vi "AO.vi"() -> ()   [LabVIEW 2023]
panel:
  out "error out":errorcluster
  in  "error in (no error)":errorcluster
  out "elements 4":variant[](array[variant])
  out "elements 3":variant[](array[variant])
  out "elements 2":variant[](array[variant])
  out "max queue size":i32
  out "# elements in queue":i32
  out "elements":variant[](array[variant])
  out "current time":timestamp
  out "overflow? 4":bool
  out "overflow? 3":bool
  out "overflow? 2":bool
  out "overflow?":bool
  out "startr_time":timestamp
  out "Waveform Chart":waveform(dbl)(graph)
  in  "Number of Samples":i32=1000
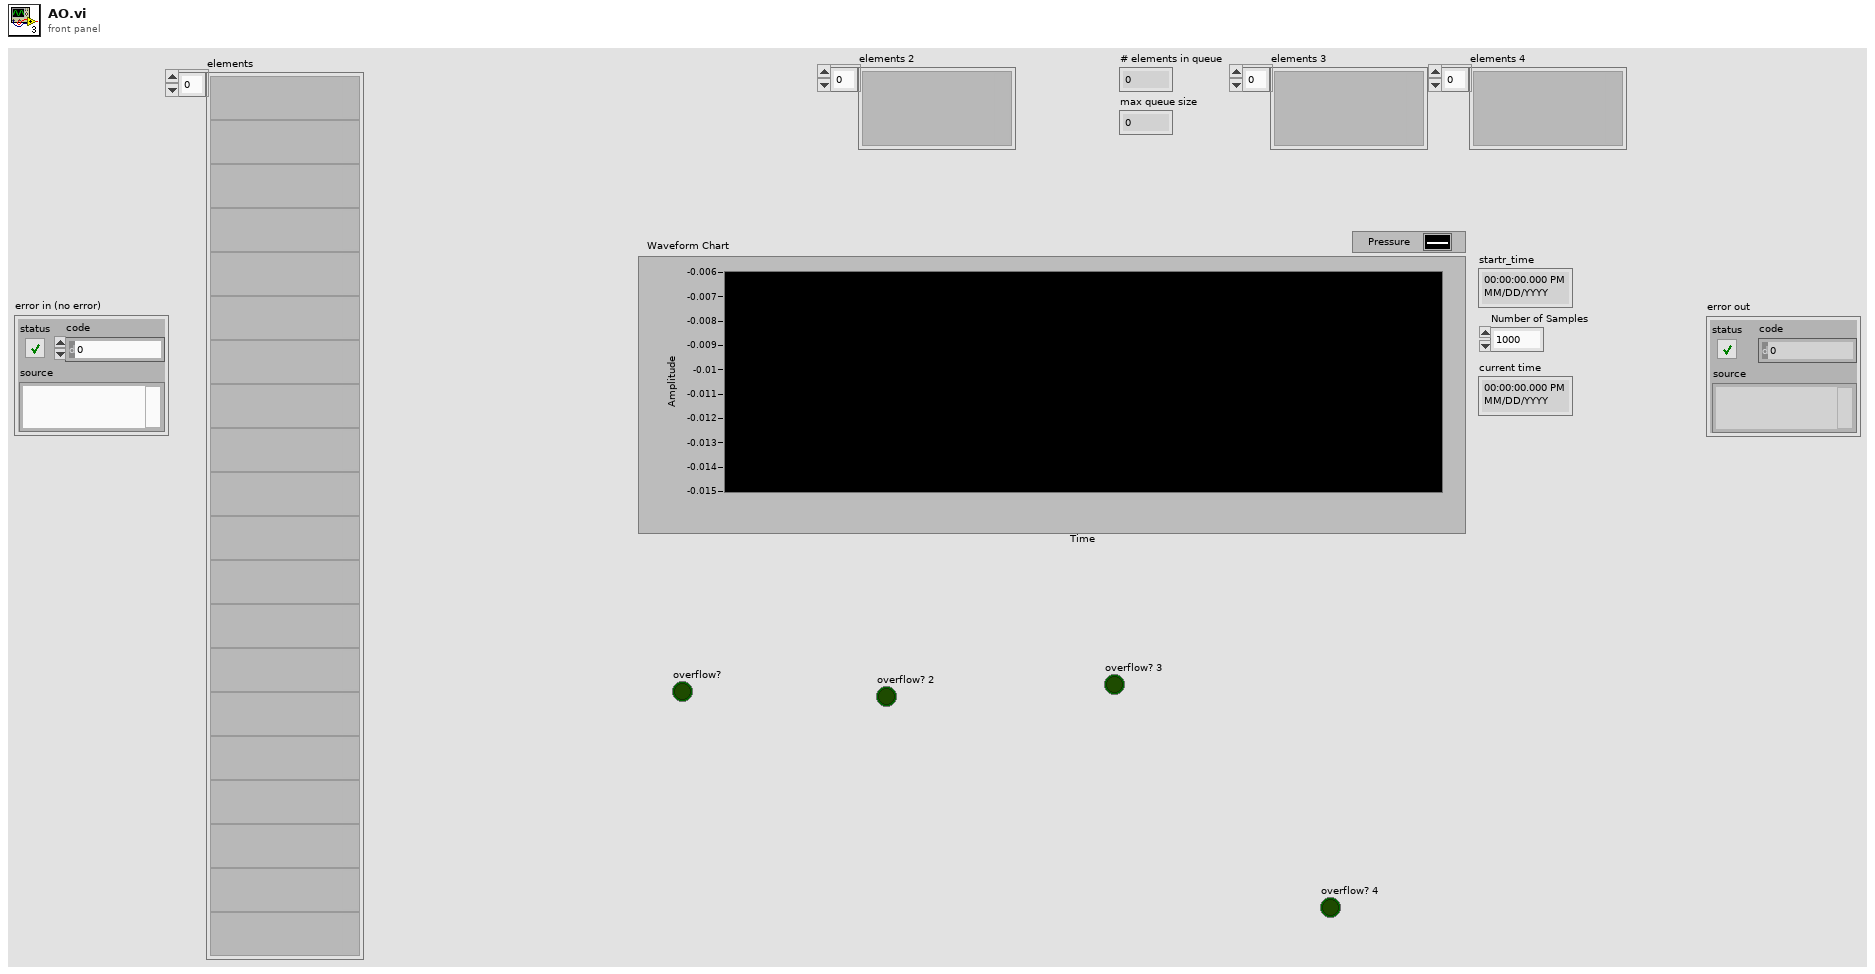
[diagram p1: front panel]
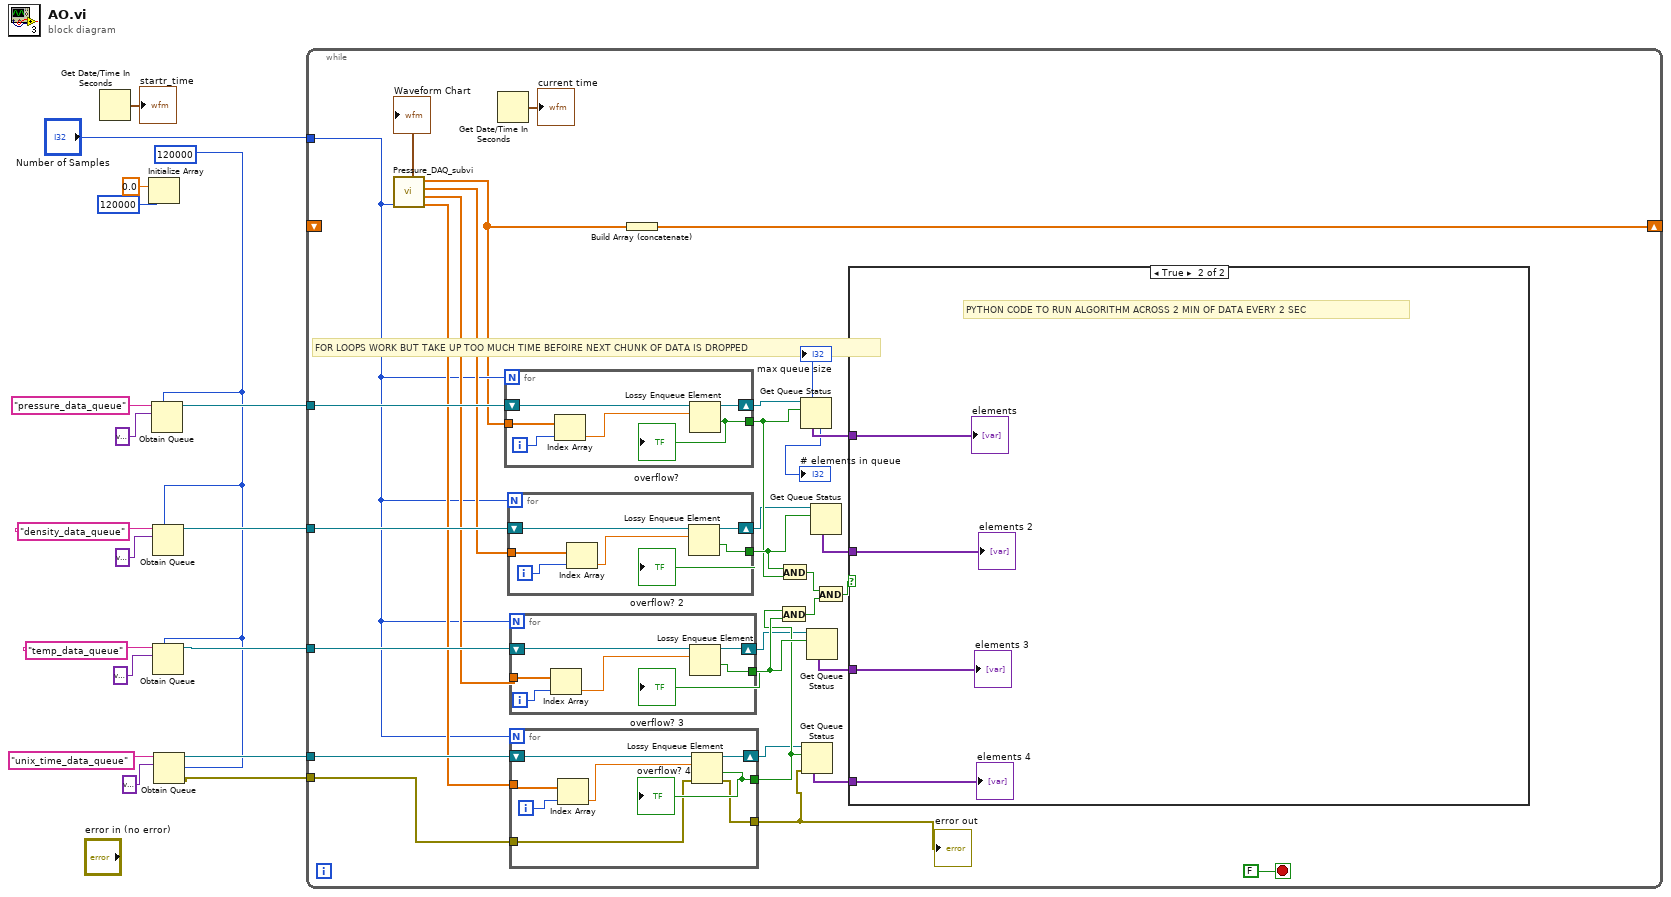
[diagram p0: block diagram]
diagram:
  w4 = 120000
  n1 = Get Date/Time In Seconds() -> (seconds since 1Jan1904=→"startr_time":timestamp)
  n2 = Initialize Array(0.0 ("element"), 120000 ("dimension size")) -> ()  [unwired: 1 out]
  n3 = Obtain Queue(max queue size (-1, unlimited)=w4, name (unnamed)="pressure_data_queue", element data type=variant) -> (queue out=w9:refnum<queue>)  [unwired: 2 in, 2 out]
  n4 = Obtain Queue(max queue size (-1, unlimited)=w4, name (unnamed)="density_data_queue", element data type=variant) -> (queue out=w8:refnum<queue>)  [unwired: 2 in, 2 out]
  n5 = Obtain Queue(max queue size (-1, unlimited)=w4, name (unnamed)="temp_data_queue", element data type=variant) -> (queue out=w7:refnum<queue>)  [unwired: 2 in, 2 out]
  n6 = Obtain Queue(max queue size (-1, unlimited)=w4, name (unnamed)="unix_time_data_queue", element data type=variant) -> (queue out=w6:refnum<queue>, error out=w1:errorcluster)  [unwired: 2 in, 1 out]
  n7 = while {
    tunnel: "Number of Samples" -> [w34]
    tunnel: w9 -> [w48]
    tunnel: w8 -> [w47]
    tunnel: w7 -> [w46]
    tunnel: w6 -> [w45]
    shift-right: [w22] -> _
    shift-left: _ -> [_]
    tunnel: w1 -> [w20]
    stop <- FALSE stop-if-true
    # "FOR LOOPS WORK BUT TAKE UP TOO MUCH TIME BEFOIRE NEXT CHUNK OF DATA IS DROPPED"
    n8 = call "Pressure_DAQ_subvi.vi"("Number of Samples"=w34) -> ("Waveform Chart"=→"Waveform Chart":waveform(dbl), "pressure_Vdc"=w21:dbl[], "density_constant"=w37:dbl[], "temp_constant"=w36:dbl[], "unix_time"=w35:dbl[])  [unwired: 5 in]
    n9 = Get Date/Time In Seconds() -> (seconds since 1Jan1904=→"current time":timestamp)
    n10 = for {
      N: w34 -> [_]
      tunnel: [w75] -> w33
      tunnel: w21 -> [w73]
      shift-right: [w74] -> w32
      shift-left: w48 -> [w76]
      i -> [w72]
      n11 = Index Array(array=w73, index=w72) -> (element=w71:dbl)
      n12 = Lossy Enqueue Element(queue=w76, element=w71) -> (queue out=w74:refnum<queue>, overflow?=w75:bool)  [unwired: 1 in, 2 out]
      "overflow?" <- w75
    }
    n13 = for {
      N: w34 -> [_]
      tunnel: [w68] -> w40
      tunnel: w37 -> [w66]
      shift-right: [w69] -> w28
      shift-left: w47 -> [w70]
      i -> [w65]
      n14 = Index Array(array=w66, index=w65) -> (element=w67:dbl)
      n15 = Lossy Enqueue Element(queue=w70, element=w67) -> (queue out=w69:refnum<queue>, overflow?=w68:bool)  [unwired: 1 in, 2 out]
      "overflow? 2" <- w68
    }
    n16 = for {
      N: w34 -> [_]
      tunnel: [w62] -> w39
      tunnel: w36 -> [w60]
      shift-right: [w63] -> w27
      shift-left: w46 -> [w64]
      i -> [w61]
      n17 = Index Array(array=w60, index=w61) -> (element=w59:dbl)
      n18 = Lossy Enqueue Element(queue=w64, element=w59) -> (queue out=w63:refnum<queue>, overflow?=w62:bool)  [unwired: 1 in, 2 out]
      "overflow? 3" <- w62
    }
    n19 = for {
      N: w34 -> [_]
      tunnel: [w56] -> w38
      tunnel: w35 -> [w54]
      shift-right: [w57] -> w26
      shift-left: w45 -> [w58]
      tunnel: [w52] -> w19
      tunnel: w20 -> [w51]
      i -> [w55]
      n20 = Index Array(array=w54, index=w55) -> (element=w53:dbl)
      n21 = Lossy Enqueue Element(queue=w58, element=w53, error in (no error)=w51) -> (queue out=w57:refnum<queue>, overflow?=w56:bool, error out=w52:errorcluster)  [unwired: 1 out]
      "overflow? 4" <- w56
    }
    "error out" <- w19
    n22 = Build Array (concatenate)(w21) -> (w22:dbl[])
    n23 = And(x=w38, y=w39) -> (x .and. y?=w44:bool)
    n24 = And(x=w40, y=w33) -> (x .and. y?=w43:bool)
    n25 = Get Queue Status(queue=w32, return elements? (F)=w33) -> (max queue size=→"max queue size":i32, # elements in queue=→"# elements in queue":i32, elements=w30:variant[])  [unwired: 1 in, 5 out]
    n26 = Get Queue Status(queue=w26, return elements? (F)=w38, error in (no error)=w19) -> (elements=w23:variant[])  [unwired: 7 out]
    n27 = Get Queue Status(queue=w27, return elements? (F)=w39) -> (elements=w24:variant[])  [unwired: 1 in, 7 out]
    n28 = Get Queue Status(queue=w28, return elements? (F)=w40) -> (elements=w25:variant[])  [unwired: 1 in, 7 out]
    n29 = And(x=w43, y=w44) -> (x .and. y?=w42:bool)
    n30 = case shown="True" w42 {
      tunnel: w30 -> [_ w80]
      tunnel: w25 -> [_ w79]
      tunnel: w24 -> [_ w78]
      tunnel: w23 -> [_ w77]
      frame False {
      }
      frame True {
        # "PYTHON CODE TO RUN ALGORITHM ACROSS 2 MIN OF DATA EVERY 2 SEC"
        "elements" <- w80
        "elements 2" <- w79
        "elements 3" <- w78
        "elements 4" <- w77
      }
    }
  }
